vi "Enqueue Write.vi"(8 "error in (no error)":errorcluster, 10 "data":waveform(cdb), 11 "disk queue":refnum<queue>) -> (0 "error out":errorcluster)   [LabVIEW 2021]
uses:
  Write Message with Waveform.ctl
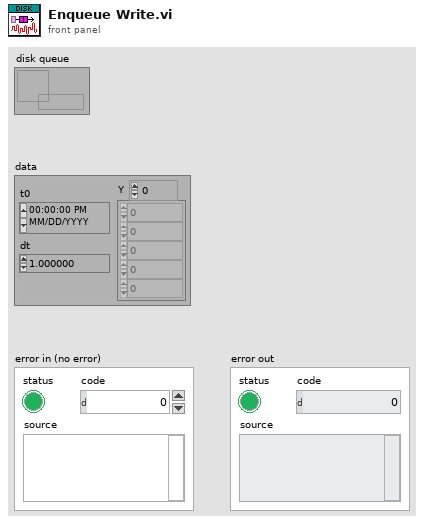
[diagram p1: front panel]
types:
  T1 = enum16{"Close TDMS", "Initialize TDMS", "Write", "Exit"}
  T2 = typedef "Write Message with Waveform.ctl" = cluster{"wfm dat":waveform(cdb), "msg":enum16{"Close TDMS", "Initialize TDMS", "Write", "Exit"}}
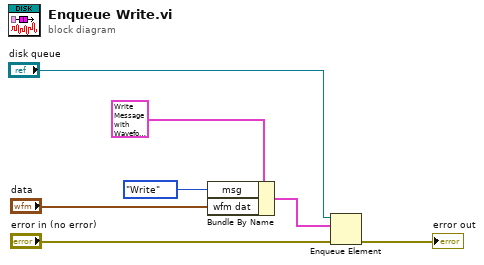
[diagram p0: block diagram]
diagram:
  n1 = Bundle By Name(cluster=T2 {"wfm dat"={"t0"=timestamp(0 s since 1904-01-01), "dt"=0.0, "Y"=[]}, "msg"=enum."Initialize TDMS"} ("element"), "msg"=T1."Write", "wfm dat"="data") -> (w7:T2)
  n2 = Enqueue Element(queue="disk queue", element=w7, error in (no error)="error in (no error)") -> (error out=→"error out":errorcluster)  [unwired: 1 in, 2 out]
